vi "Tree.vi"   [LabVIEW 2013]
uses:
  StructureTypes.ctl
panel:
  # "This doesn't do anything..."
types:
  T1 = typedef "StructureTypes.ctl" = enum16{"CaseStructure", "EventStructure"}
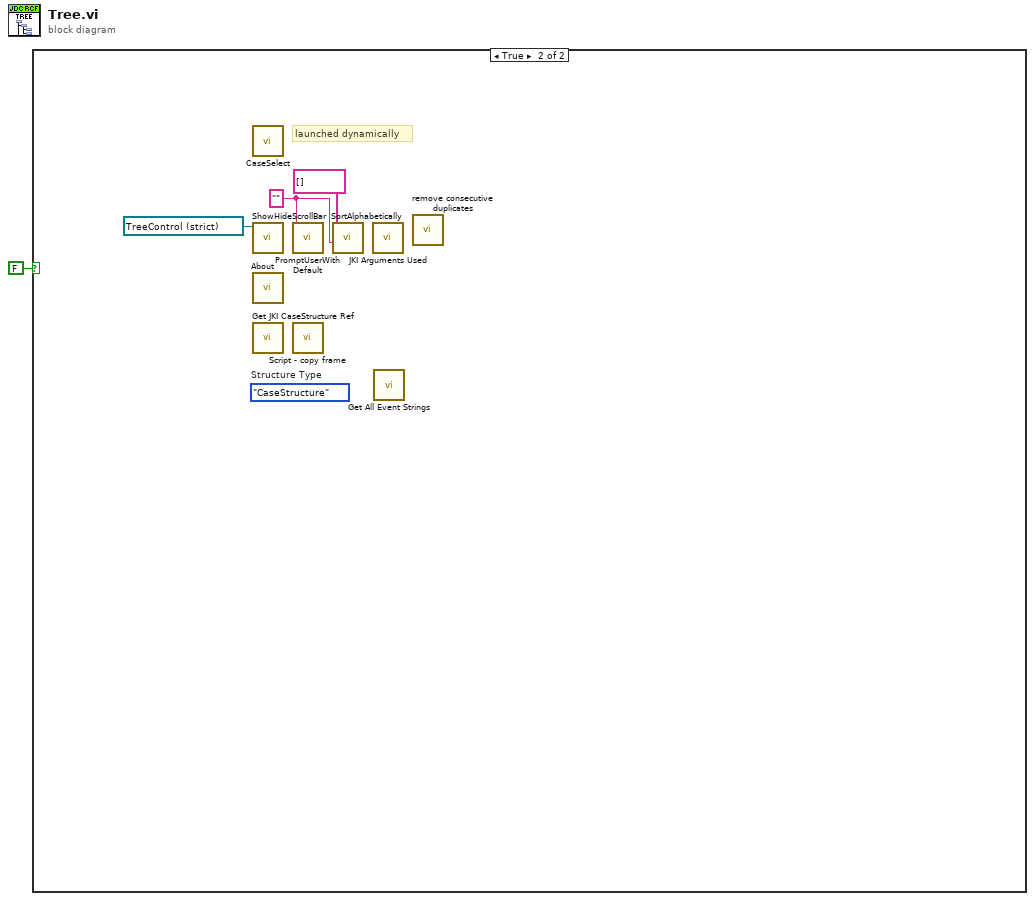
[diagram p0: block diagram]
diagram:
  n1 = case shown="True" FALSE {
    frame False {
    }
    frame True {
      w2 = "" ("SectHdr")
      (unwired) StructureTypes."CaseStructure"  # Structure Type
      # "launched dynamically"
      n2 = call "CaseSelect.vi"() -> ()  [unwired: 12 in]
      n3 = call "ShowHideScrollBar.vi"("reference"=refnum<vi> refnum) -> ()  [unwired: 7 in, 4 out]
      n4 = call "About.vi"() -> ()  [unwired: 1 in]
      n5 = call "Get JKI CaseStructure Ref.vi"() -> ()  [unwired: 9 in, 3 out]
      n6 = call "PromptUserWithDefault.vi"("Section"=w2) -> ()  [unwired: 9 in, 2 out]
      n7 = call "Script - copy frame.vi"() -> ()  [unwired: 11 in, 1 out]
      n8 = call "SortAlphabetically.vi"("TreeSectHdrs"=w2, "FrameNames"=string[] []) -> ()  [unwired: 8 in, 2 out]
      n9 = call "JKI Arguments Used.vi"() -> ()  [unwired: 10 in, 2 out]
      n10 = call "Get All Event Strings.vi"() -> ()  [unwired: 9 in, 3 out]
      n11 = call "remove consecutive duplicates.vi"() -> ()  [unwired: 11 in, 1 out]
    }
  }
